vi "Send Operator_Name.vi"(8 "error in":errorcluster, 10 "Operator Name":string, 11 "Engine in":refnum<class "Engine.lvclass">) -> (0 "error out":errorcluster, 3 "Engine out":refnum<class "Engine.lvclass">)   [LabVIEW 2019, in "Engine.lvlib" / "Engine.lvclass"]
doc: "Trigger the Update Operator Name Event (allowing components to update any references to the operator name)"
uses:
  Project/Engine.lvclass
  Project/Engine.lvclass/Engine.ctl
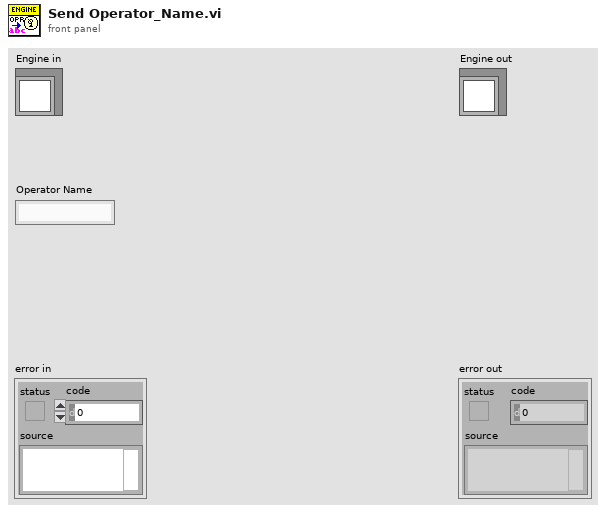
[diagram p1: front panel]
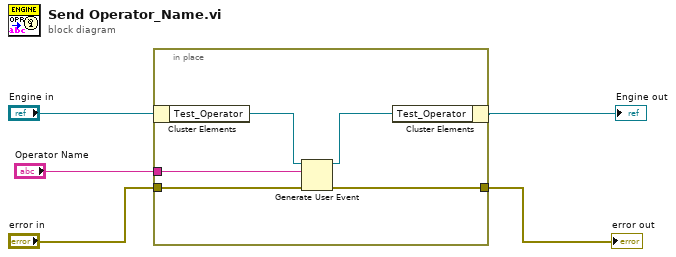
[diagram p0: block diagram]
diagram:
  n1 = in-place {
    in-place-border: "error in" -> [w8]
    in-place-border: [w7] -> w2
    in-place-border: "Operator Name" -> [w6]
    n2 = in-place-cluster #1("Engine in") -> ("Test_Operator"=w10:refnum<user-event>)
    n3 = Generate User Event(user event=w10, event data cluster=w6, error in=w8) -> (user event out=w9:refnum<user-event>, error out=w7:errorcluster)  [unwired: 1 in]
    n4 = in-place-cluster #1("Test_Operator"=w9) -> (→"Engine out":refnum<class "Engine.lvclass">)
  }
  "error out" <- w2
